vi "Test Phase Retrieval.vi"() -> ()   [LabVIEW 2018]
uses:
  File IO/Image/Tiff/Tiff reader.lvlib
panel:
  out "Function name":string
  out "Python file":path
  out "error out":errorcluster={"status"=FALSE, "code"=0, "source"="XXX"}
  out "Image path":path
  out "Pupil Graph":dbl[][](graph)
  out "Module parent folder":path
  out "Stack sizes":i32[](array[numeric])
  out "Stack Preview":u16[][](graph)
  in  "Slice to preview":i32(slide) scale=0.0..13.0
  # "From python code:"
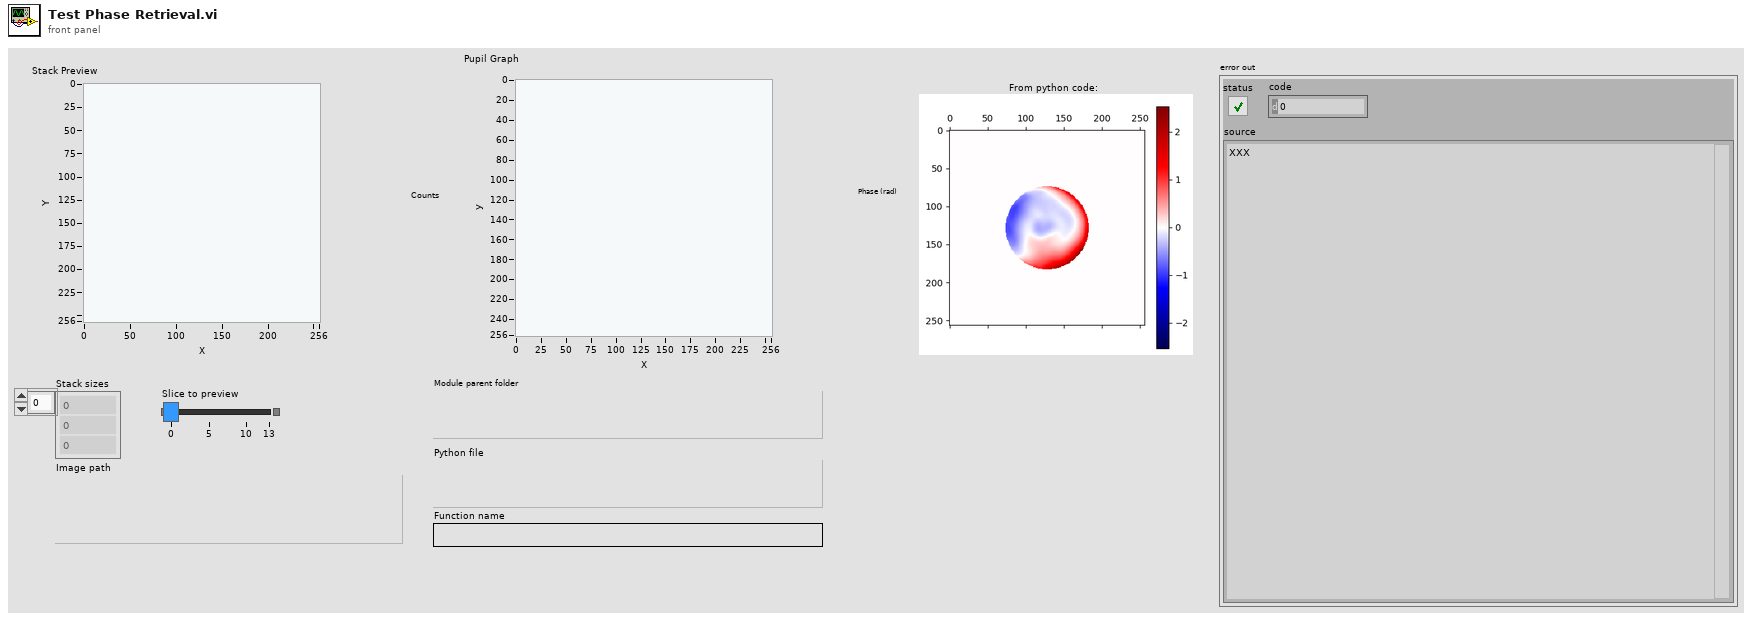
[diagram p1: front panel]
types:
  T1 = enum32{"Gray", "Binary", "Gradient", "Rainbow", "Temperature"}
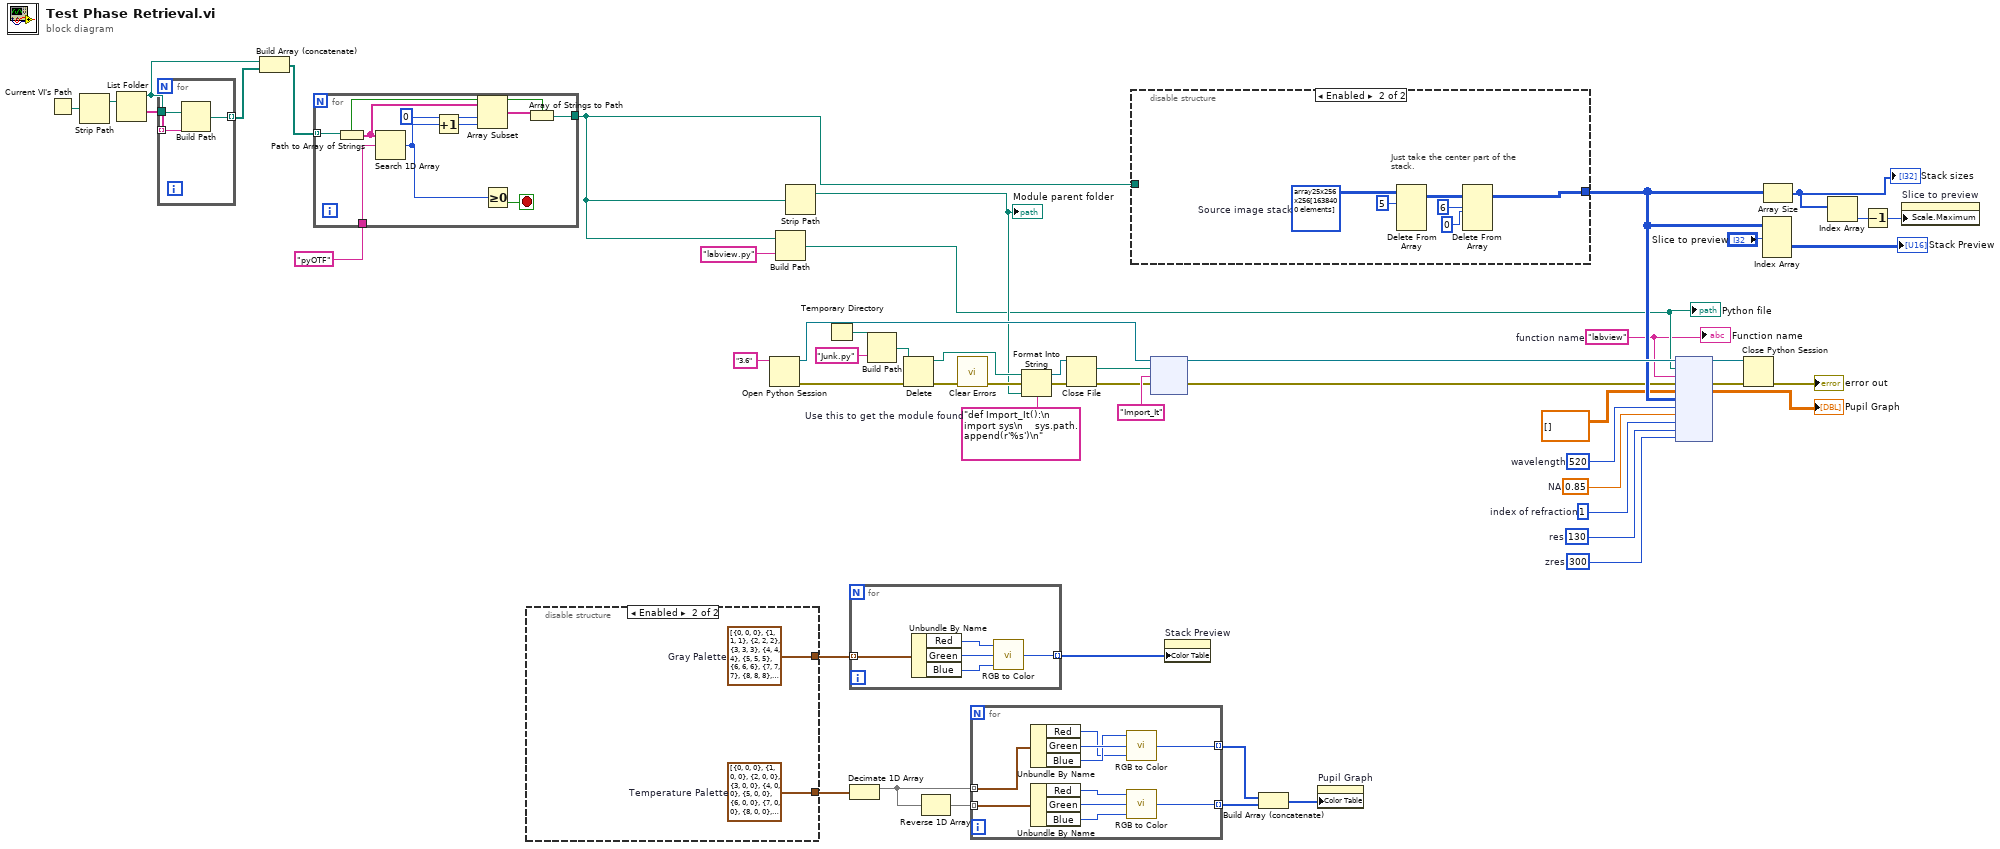
[diagram p0: block diagram]
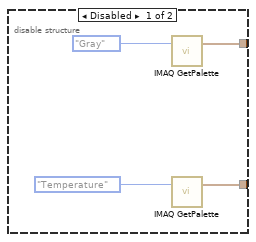
[diagram p2: hidden frame]
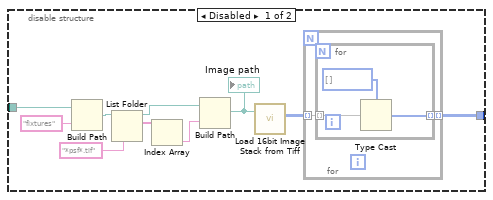
[diagram p3: hidden frame]
diagram:
  w27 = 1  # index of refraction
  w37 = "def Import_It():\n    import sys\n    sys.path.append(r'%s')\n"  # Use this to get the module found
  w26 = 300  # zres
  w25 = 130  # res
  w38 = 0.85  # NA
  w39 = 520  # wavelength
  w2 = "labview"  # function name
  n1 = Current VI's Path() -> (path=w11:path)
  n2 = Strip Path(path=w11) -> (stripped path=w10:path)  [unwired: 1 out]
  n3 = List Folder(path=w10) -> (path out=w7:path, folder names=w9:string[])  [unwired: 3 in, 2 out]
  n4 = for {
    tunnel: w9 -> [w55] mode=indexing
    tunnel: w7 -> [w54]
    tunnel: [w53] -> w8 mode=indexing
    n5 = Build Path(base path=w54, name or relative path=w55) -> (appended path=w53:path)
  }
  n6 = Build Array (concatenate)(w7, w8) -> (w6:path[])
  n7 = for {
    tunnel: w6 -> [w65] mode=indexing
    tunnel: "pyOTF" ("name or relative path") -> [w64]
    tunnel: [w57] -> w4
    stop <- w63 stop-if-true
    n8 = Path to Array of Strings(0:w65) -> (1:w58:bool, 2:w62:string[])
    n9 = Search 1D Array(1D array=w62, element=w64) -> (index of element=w61:i32)  [unwired: 1 in]
    n10 = Increment(x=w61) -> (x+1=w56:i32)
    n11 = Array Subset(array=w62, index=0, length=w56) -> (w59:string[])
    n12 = Greater Or Equal To 0?(x=w61) -> (x >= 0?=w63:bool)
    n13 = Array of Strings to Path(0:w59, 1:w58) -> (2:w57:path)
  }
  n14 = disable-structure shown="Enabled" {
    disable-tunnel: [w68 w71] -> w52
    disable-tunnel: [w66 w70] -> w19
    frame Disabled {
      n15 = call "IMAQ GetPalette"("Palette Number (gray)"=T1."Gray") -> ("Color Palette"=w66:cluster{"Red":u8, "Green":u8, "Blue":u8}[])  [unwired: 4 in, 1 out]
      n16 = call "IMAQ GetPalette"("Palette Number (gray)"=T1."Temperature" ("Palette E")) -> ("Color Palette"=w68:cluster{"Red":u8, "Green":u8, "Blue":u8}[])  [unwired: 4 in, 1 out]
    }
    frame Enabled {
      w70 = cluster{"Red":u8, "Green":u8, "Blue":u8}[] [{"Red"=0, "Green"=0, "Blue"=0}, {"Red"=1, "Green"=1, "Blue"=1}, {"Red"=2, "Green"=2, "Blue"=2}, {"Red"=3, "Green"=3, "Blue"=3}, {"Red"=4, "Green"=4, "Blue"=4}, {"Red"=5, "Green"=5, "Blue"=5}, {"Red"=6, "Green"=6, "Blue"=6}, {"Red"=7, "Green"=7, "Blue"=7}, {"Red"=8, "Green"=8, "Blue"=8}, {"Red"=9, "Green"=9, "Blue"=9}, {"Red"=10, "Green"=10, "Blue"=10}, {"Red"=11, "Green"=11, "Blue"=11}, {"Red"=12, "Green"=12, "Blue"=12}, {"Red"=13, "Green"=13, "Blue"=13}, {"Red"=14, "Green"=14, "Blue"=14}, {"Red"=15, "Green"=15, "Blue"=15}, {"Red"=16, "Green"=16, "Blue"=16}, {"Red"=17, "Green"=17, "Blue"=17}, {"Red"=18, "Green"=18, "Blue"=18}, {"Red"=19, "Green"=19, "Blue"=19}, {"Red"=20, "Green"=20, "Blue"=20}, {"Red"=21, "Green"=21, "Blue"=21}, {"Red"=22, "Green"=22, "Blue"=22}, {"Red"=23, "Green"=23, "Blue"=23}, {"Red"=24, "Green"=24, "Blue"=24}, {"Red"=25, "Green"=25, "Blue"=25}, {"Red"=26, "Green"=26, "Blue"=26}, {"Red"=27, "Green"=27, "Blue"=27}, {"Red"=28, "Green"=28, "Blue"=28}, {"Red"=29, "Green"=29, "Blue"=29}, {"Red"=30, "Green"=30, "Blue"=30}, {"Red"=31, "Green"=31, "Blue"=31}, {"Red"=32, "Green"=32, "Blue"=32}, {"Red"=33, "Green"=33, "Blue"=33}, {"Red"=34, "Green"=34, "Blue"=34}, {"Red"=35, "Green"=35, "Blue"=35}, {"Red"=36, "Green"=36, "Blue"=36}, {"Red"=37, "Green"=37, "Blue"=37}, {"Red"=38, "Green"=38, "Blue"=38}, {"Red"=39, "Green"=39, "Blue"=39}, {"Red"=40, "Green"=40, "Blue"=40}, {"Red"=41, "Green"=41, "Blue"=41}, {"Red"=42, "Green"=42, "Blue"=42}, {"Red"=43, "Green"=43, "Blue"=43}, {"Red"=44, "Green"=44, "Blue"=44}, {"Red"=45, "Green"=45, "Blue"=45}, {"Red"=46, "Green"=46, "Blue"=46}, {"Red"=47, "Green"=47, "Blue"=47}, {"Red"=48, "Green"=48, "Blue"=48}, {"Red"=49, "Green"=49, "Blue"=49}, {"Red"=50, "Green"=50, "Blue"=50}, {"Red"=51, "Green"=51, "Blue"=51}, {"Red"=52, "Green"=52, "Blue"=52}, {"Red"=53, "Green"=53, "Blue"=53}, {"Red"=54, "Green"=54, "Blue"=54}, {"Red"=55, "Green"=55, "Blue"=55}, {"Red"=56, "Green"=56, "Blue"=56}, {"Red"=57, "Green"=57, "Blue"=57}, {"Red"=58, "Green"=58, "Blue"=58}, {"Red"=59, "Green"=59, "Blue"=59}, {"Red"=60, "Green"=60, "Blue"=60}, {"Red"=61, "Green"=61, "Blue"=61}, {"Red"=62, "Green"=62, "Blue"=62}, {"Red"=63, "Green"=63, "Blue"=63}, {"Red"=64, "Green"=64, "Blue"=64}, {"Red"=65, "Green"=65, "Blue"=65}, {"Red"=66, "Green"=66, "Blue"=66}, {"Red"=67, "Green"=67, "Blue"=67}, {"Red"=68, "Green"=68, "Blue"=68}, {"Red"=69, "Green"=69, "Blue"=69}, {"Red"=70, "Green"=70, "Blue"=70}, {"Red"=71, "Green"=71, "Blue"=71}, {"Red"=72, "Green"=72, "Blue"=72}, {"Red"=73, "Green"=73, "Blue"=73}, {"Red"=74, "Green"=74, "Blue"=74}, {"Red"=75, "Green"=75, "Blue"=75}, {"Red"=76, "Green"=76, "Blue"=76}, {"Red"=77, "Green"=77, "Blue"=77}, {"Red"=78, "Green"=78, "Blue"=78}, {"Red"=79, "Green"=79, "Blue"=79}, {"Red"=80, "Green"=80, "Blue"=80}, {"Red"=81, "Green"=81, "Blue"=81}, {"Red"=82, "Green"=82, "Blue"=82}, {"Red"=83, "Green"=83, "Blue"=83}, {"Red"=84, "Green"=84, "Blue"=84}, {"Red"=85, "Green"=85, "Blue"=85}, {"Red"=86, "Green"=86, "Blue"=86}, {"Red"=87, "Green"=87, "Blue"=87}, {"Red"=88, "Green"=88, "Blue"=88}, {"Red"=89, "Green"=89, "Blue"=89}, {"Red"=90, "Green"=90, "Blue"=90}, {"Red"=91, "Green"=91, "Blue"=91}, {"Red"=92, "Green"=92, "Blue"=92}, {"Red"=93, "Green"=93, "Blue"=93}, {"Red"=94, "Green"=94, "Blue"=94}, {"Red"=95, "Green"=95, "Blue"=95}, {"Red"=96, "Green"=96, "Blue"=96}, {"Red"=97, "Green"=97, "Blue"=97}, {"Red"=98, "Green"=98, "Blue"=98}, {"Red"=99, "Green"=99, "Blue"=99}, {"Red"=100, "Green"=100, "Blue"=100}, {"Red"=101, "Green"=101, "Blue"=101}, {"Red"=102, "Green"=102, "Blue"=102}, {"Red"=103, "Green"=103, "Blue"=103}, {"Red"=104, "Green"=104, "Blue"=104}, {"Red"=105, "Green"=105, "Blue"=105}, {"Red"=106, "Green"=106, "Blue"=106}, {"Red"=107, "Green"=107, "Blue"=107}, {"Red"=108, "Green"=108, "Blue"=108}, {"Red"=109, "Green"=109, "Blue"=109}, {"Red"=110, "Green"=110, "Blue"=110}, {"Red"=111, "Green"=111, "Blue"=111}, {"Red"=112, "Green"=112, "Blue"=112}, {"Red"=113, "Green"=113, "Blue"=113}, {"Red"=114, "Green"=114, "Blue"=114}, {"Red"=115, "Green"=115, "Blue"=115}, {"Red"=116, "Green"=116, "Blue"=116}, {"Red"=117, "Green"=117, "Blue"=117}, {"Red"=118, "Green"=118, "Blue"=118}, {"Red"=119, "Green"=119, "Blue"=119}, {"Red"=120, "Green"=120, "Blue"=120}, {"Red"=121, "Green"=121, "Blue"=121}, {"Red"=122, "Green"=122, "Blue"=122}, {"Red"=123, "Green"=123, "Blue"=123}, {"Red"=124, "Green"=124, "Blue"=124}, {"Red"=125, "Green"=125, "Blue"=125}, {"Red"=126, "Green"=126, "Blue"=126}, {"Red"=127, "Green"=127, "Blue"=127}, {"Red"=128, "Green"=128, "Blue"=128}, {"Red"=129, "Green"=129, "Blue"=129}, {"Red"=130, "Green"=130, "Blue"=130}, {"Red"=131, "Green"=131, "Blue"=131}, {"Red"=132, "Green"=132, "Blue"=132}, {"Red"=133, "Green"=133, "Blue"=133}, {"Red"=134, "Green"=134, "Blue"=134}, {"Red"=135, "Green"=135, "Blue"=135}, {"Red"=136, "Green"=136, "Blue"=136}, {"Red"=137, "Green"=137, "Blue"=137}, {"Red"=138, "Green"=138, "Blue"=138}, {"Red"=139, "Green"=139, "Blue"=139}, {"Red"=140, "Green"=140, "Blue"=140}, {"Red"=141, "Green"=141, "Blue"=141}, {"Red"=142, "Green"=142, "Blue"=142}, {"Red"=143, "Green"=143, "Blue"=143}, {"Red"=144, "Green"=144, "Blue"=144}, {"Red"=145, "Green"=145, "Blue"=145}, {"Red"=146, "Green"=146, "Blue"=146}, {"Red"=147, "Green"=147, "Blue"=147}, {"Red"=148, "Green"=148, "Blue"=148}, {"Red"=149, "Green"=149, "Blue"=149}, {"Red"=150, "Green"=150, "Blue"=150}, {"Red"=151, "Green"=151, "Blue"=151}, {"Red"=152, "Green"=152, "Blue"=152}, {"Red"=153, "Green"=153, "Blue"=153}, {"Red"=154, "Green"=154, "Blue"=154}, {"Red"=155, "Green"=155, "Blue"=155}, {"Red"=156, "Green"=156, "Blue"=156}, {"Red"=157, "Green"=157, "Blue"=157}, {"Red"=158, "Green"=158, "Blue"=158}, {"Red"=159, "Green"=159, "Blue"=159}, {"Red"=160, "Green"=160, "Blue"=160}, {"Red"=161, "Green"=161, "Blue"=161}, {"Red"=162, "Green"=162, "Blue"=162}, {"Red"=163, "Green"=163, "Blue"=163}, {"Red"=164, "Green"=164, "Blue"=164}, {"Red"=165, "Green"=165, "Blue"=165}, {"Red"=166, "Green"=166, "Blue"=166}, {"Red"=167, "Green"=167, "Blue"=167}, {"Red"=168, "Green"=168, "Blue"=168}, {"Red"=169, "Green"=169, "Blue"=169}, {"Red"=170, "Green"=170, "Blue"=170}, {"Red"=171, "Green"=171, "Blue"=171}, {"Red"=172, "Green"=172, "Blue"=172}, {"Red"=173, "Green"=173, "Blue"=173}, {"Red"=174, "Green"=174, "Blue"=174}, {"Red"=175, "Green"=175, "Blue"=175}, {"Red"=176, "Green"=176, "Blue"=176}, {"Red"=177, "Green"=177, "Blue"=177}, {"Red"=178, "Green"=178, "Blue"=178}, {"Red"=179, "Green"=179, "Blue"=179}, {"Red"=180, "Green"=180, "Blue"=180}, {"Red"=181, "Green"=181, "Blue"=181}, {"Red"=182, "Green"=182, "Blue"=182}, {"Red"=183, "Green"=183, "Blue"=183}, {"Red"=184, "Green"=184, "Blue"=184}, {"Red"=185, "Green"=185, "Blue"=185}, {"Red"=186, "Green"=186, "Blue"=186}, {"Red"=187, "Green"=187, "Blue"=187}, {"Red"=188, "Green"=188, "Blue"=188}, {"Red"=189, "Green"=189, "Blue"=189}, {"Red"=190, "Green"=190, "Blue"=190}, {"Red"=191, "Green"=191, "Blue"=191}, {"Red"=192, "Green"=192, "Blue"=192}, {"Red"=193, "Green"=193, "Blue"=193}, {"Red"=194, "Green"=194, "Blue"=194}, {"Red"=195, "Green"=195, "Blue"=195}, {"Red"=196, "Green"=196, "Blue"=196}, {"Red"=197, "Green"=197, "Blue"=197}, {"Red"=198, "Green"=198, "Blue"=198}, {"Red"=199, "Green"=199, "Blue"=199}, {"Red"=200, "Green"=200, "Blue"=200}, {"Red"=201, "Green"=201, "Blue"=201}, {"Red"=202, "Green"=202, "Blue"=202}, {"Red"=203, "Green"=203, "Blue"=203}, {"Red"=204, "Green"=204, "Blue"=204}, {"Red"=205, "Green"=205, "Blue"=205}, {"Red"=206, "Green"=206, "Blue"=206}, {"Red"=207, "Green"=207, "Blue"=207}, {"Red"=208, "Green"=208, "Blue"=208}, {"Red"=209, "Green"=209, "Blue"=209}, {"Red"=210, "Green"=210, "Blue"=210}, {"Red"=211, "Green"=211, "Blue"=211}, {"Red"=212, "Green"=212, "Blue"=212}, {"Red"=213, "Green"=213, "Blue"=213}, {"Red"=214, "Green"=214, "Blue"=214}, {"Red"=215, "Green"=215, "Blue"=215}, {"Red"=216, "Green"=216, "Blue"=216}, {"Red"=217, "Green"=217, "Blue"=217}, {"Red"=218, "Green"=218, "Blue"=218}, {"Red"=219, "Green"=219, "Blue"=219}, {"Red"=220, "Green"=220, "Blue"=220}, {"Red"=221, "Green"=221, "Blue"=221}, {"Red"=222, "Green"=222, "Blue"=222}, {"Red"=223, "Green"=223, "Blue"=223}, {"Red"=224, "Green"=224, "Blue"=224}, {"Red"=225, "Green"=225, "Blue"=225}, {"Red"=226, "Green"=226, "Blue"=226}, {"Red"=227, "Green"=227, "Blue"=227}, {"Red"=228, "Green"=228, "Blue"=228}, {"Red"=229, "Green"=229, "Blue"=229}, {"Red"=230, "Green"=230, "Blue"=230}, {"Red"=231, "Green"=231, "Blue"=231}, {"Red"=232, "Green"=232, "Blue"=232}, {"Red"=233, "Green"=233, "Blue"=233}, {"Red"=234, "Green"=234, "Blue"=234}, {"Red"=235, "Green"=235, "Blue"=235}, {"Red"=236, "Green"=236, "Blue"=236}, {"Red"=237, "Green"=237, "Blue"=237}, {"Red"=238, "Green"=238, "Blue"=238}, {"Red"=239, "Green"=239, "Blue"=239}, {"Red"=240, "Green"=240, "Blue"=240}, {"Red"=241, "Green"=241, "Blue"=241}, {"Red"=242, "Green"=242, "Blue"=242}, {"Red"=243, "Green"=243, "Blue"=243}, {"Red"=244, "Green"=244, "Blue"=244}, {"Red"=245, "Green"=245, "Blue"=245}, {"Red"=246, "Green"=246, "Blue"=246}, {"Red"=247, "Green"=247, "Blue"=247}, {"Red"=248, "Green"=248, "Blue"=248}, {"Red"=249, "Green"=249, "Blue"=249}, {"Red"=250, "Green"=250, "Blue"=250}, {"Red"=251, "Green"=251, "Blue"=251}, {"Red"=252, "Green"=252, "Blue"=252}, {"Red"=253, "Green"=253, "Blue"=253}, {"Red"=254, "Green"=254, "Blue"=254}, {"Red"=255, "Green"=255, "Blue"=255}]  # Gray Palette
      w71 = cluster{"Red":u8, "Green":u8, "Blue":u8}[] [{"Red"=0, "Green"=0, "Blue"=0}, {"Red"=1, "Green"=0, "Blue"=0}, {"Red"=2, "Green"=0, "Blue"=0}, {"Red"=3, "Green"=0, "Blue"=0}, {"Red"=4, "Green"=0, "Blue"=0}, {"Red"=5, "Green"=0, "Blue"=0}, {"Red"=6, "Green"=0, "Blue"=0}, {"Red"=7, "Green"=0, "Blue"=0}, {"Red"=8, "Green"=0, "Blue"=0}, {"Red"=9, "Green"=0, "Blue"=0}, {"Red"=10, "Green"=0, "Blue"=0}, {"Red"=11, "Green"=0, "Blue"=0}, {"Red"=12, "Green"=0, "Blue"=0}, {"Red"=13, "Green"=0, "Blue"=0}, {"Red"=14, "Green"=0, "Blue"=0}, {"Red"=15, "Green"=0, "Blue"=0}, {"Red"=16, "Green"=0, "Blue"=0}, {"Red"=17, "Green"=0, "Blue"=0}, {"Red"=18, "Green"=0, "Blue"=0}, {"Red"=19, "Green"=0, "Blue"=0}, {"Red"=20, "Green"=0, "Blue"=0}, {"Red"=21, "Green"=0, "Blue"=0}, {"Red"=22, "Green"=0, "Blue"=0}, {"Red"=23, "Green"=0, "Blue"=0}, {"Red"=24, "Green"=0, "Blue"=0}, {"Red"=25, "Green"=0, "Blue"=0}, {"Red"=26, "Green"=0, "Blue"=0}, {"Red"=27, "Green"=0, "Blue"=0}, {"Red"=28, "Green"=0, "Blue"=0}, {"Red"=29, "Green"=0, "Blue"=0}, {"Red"=30, "Green"=0, "Blue"=0}, {"Red"=31, "Green"=0, "Blue"=0}, {"Red"=32, "Green"=0, "Blue"=0}, {"Red"=33, "Green"=0, "Blue"=0}, {"Red"=34, "Green"=0, "Blue"=0}, {"Red"=35, "Green"=0, "Blue"=0}, {"Red"=36, "Green"=0, "Blue"=0}, {"Red"=37, "Green"=0, "Blue"=0}, {"Red"=38, "Green"=0, "Blue"=0}, {"Red"=39, "Green"=0, "Blue"=0}, {"Red"=40, "Green"=0, "Blue"=0}, {"Red"=41, "Green"=0, "Blue"=0}, {"Red"=42, "Green"=0, "Blue"=0}, {"Red"=43, "Green"=0, "Blue"=0}, {"Red"=44, "Green"=0, "Blue"=0}, {"Red"=45, "Green"=0, "Blue"=0}, {"Red"=46, "Green"=0, "Blue"=0}, {"Red"=47, "Green"=0, "Blue"=0}, {"Red"=48, "Green"=0, "Blue"=0}, {"Red"=49, "Green"=0, "Blue"=0}, {"Red"=50, "Green"=0, "Blue"=0}, {"Red"=51, "Green"=0, "Blue"=0}, {"Red"=52, "Green"=0, "Blue"=0}, {"Red"=53, "Green"=0, "Blue"=0}, {"Red"=54, "Green"=0, "Blue"=0}, {"Red"=55, "Green"=0, "Blue"=0}, {"Red"=56, "Green"=0, "Blue"=0}, {"Red"=57, "Green"=0, "Blue"=0}, {"Red"=58, "Green"=0, "Blue"=0}, {"Red"=59, "Green"=0, "Blue"=0}, {"Red"=60, "Green"=0, "Blue"=0}, {"Red"=61, "Green"=0, "Blue"=0}, {"Red"=62, "Green"=0, "Blue"=0}, {"Red"=63, "Green"=0, "Blue"=0}, {"Red"=64, "Green"=0, "Blue"=0}, {"Red"=65, "Green"=0, "Blue"=0}, {"Red"=66, "Green"=0, "Blue"=0}, {"Red"=67, "Green"=0, "Blue"=0}, {"Red"=68, "Green"=0, "Blue"=0}, {"Red"=69, "Green"=0, "Blue"=0}, {"Red"=70, "Green"=0, "Blue"=0}, {"Red"=71, "Green"=0, "Blue"=0}, {"Red"=72, "Green"=0, "Blue"=0}, {"Red"=73, "Green"=0, "Blue"=0}, {"Red"=74, "Green"=0, "Blue"=0}, {"Red"=75, "Green"=0, "Blue"=0}, {"Red"=76, "Green"=0, "Blue"=0}, {"Red"=77, "Green"=0, "Blue"=0}, {"Red"=78, "Green"=0, "Blue"=0}, {"Red"=79, "Green"=0, "Blue"=0}, {"Red"=80, "Green"=0, "Blue"=0}, {"Red"=81, "Green"=0, "Blue"=0}, {"Red"=82, "Green"=0, "Blue"=0}, {"Red"=83, "Green"=0, "Blue"=0}, {"Red"=84, "Green"=0, "Blue"=0}, {"Red"=85, "Green"=0, "Blue"=0}, {"Red"=86, "Green"=0, "Blue"=0}, {"Red"=87, "Green"=0, "Blue"=0}, {"Red"=88, "Green"=0, "Blue"=0}, {"Red"=89, "Green"=0, "Blue"=0}, {"Red"=90, "Green"=0, "Blue"=0}, {"Red"=91, "Green"=0, "Blue"=0}, {"Red"=92, "Green"=0, "Blue"=0}, {"Red"=93, "Green"=0, "Blue"=0}, {"Red"=94, "Green"=0, "Blue"=0}, {"Red"=95, "Green"=0, "Blue"=0}, {"Red"=96, "Green"=0, "Blue"=0}, {"Red"=97, "Green"=0, "Blue"=0}, {"Red"=98, "Green"=0, "Blue"=0}, {"Red"=99, "Green"=0, "Blue"=0}, {"Red"=100, "Green"=0, "Blue"=0}, {"Red"=101, "Green"=0, "Blue"=0}, {"Red"=102, "Green"=0, "Blue"=0}, {"Red"=103, "Green"=0, "Blue"=0}, {"Red"=104, "Green"=0, "Blue"=0}, {"Red"=105, "Green"=1, "Blue"=0}, {"Red"=106, "Green"=3, "Blue"=0}, {"Red"=107, "Green"=5, "Blue"=0}, {"Red"=108, "Green"=6, "Blue"=0}, {"Red"=109, "Green"=8, "Blue"=0}, {"Red"=110, "Green"=10, "Blue"=0}, {"Red"=111, "Green"=11, "Blue"=0}, {"Red"=112, "Green"=13, "Blue"=0}, {"Red"=113, "Green"=15, "Blue"=0}, {"Red"=114, "Green"=16, "Blue"=0}, {"Red"=115, "Green"=18, "Blue"=0}, {"Red"=116, "Green"=20, "Blue"=0}, {"Red"=117, "Green"=21, "Blue"=0}, {"Red"=118, "Green"=23, "Blue"=0}, {"Red"=119, "Green"=25, "Blue"=0}, {"Red"=120, "Green"=27, "Blue"=0}, {"Red"=121, "Green"=28, "Blue"=0}, {"Red"=122, "Green"=30, "Blue"=0}, {"Red"=123, "Green"=32, "Blue"=0}, {"Red"=124, "Green"=33, "Blue"=0}, {"Red"=125, "Green"=35, "Blue"=0}, {"Red"=126, "Green"=37, "Blue"=0}, {"Red"=127, "Green"=38, "Blue"=0}, {"Red"=128, "Green"=40, "Blue"=0}, {"Red"=129, "Green"=42, "Blue"=0}, {"Red"=130, "Green"=43, "Blue"=0}, {"Red"=131, "Green"=45, "Blue"=0}, {"Red"=132, "Green"=47, "Blue"=0}, {"Red"=133, "Green"=48, "Blue"=0}, {"Red"=134, "Green"=50, "Blue"=0}, {"Red"=135, "Green"=52, "Blue"=0}, {"Red"=136, "Green"=54, "Blue"=0}, {"Red"=137, "Green"=55, "Blue"=0}, {"Red"=138, "Green"=57, "Blue"=0}, {"Red"=139, "Green"=59, "Blue"=0}, {"Red"=140, "Green"=60, "Blue"=0}, {"Red"=141, "Green"=62, "Blue"=0}, {"Red"=142, "Green"=64, "Blue"=0}, {"Red"=143, "Green"=65, "Blue"=2}, {"Red"=144, "Green"=67, "Blue"=4}, {"Red"=145, "Green"=69, "Blue"=6}, {"Red"=146, "Green"=70, "Blue"=9}, {"Red"=147, "Green"=72, "Blue"=11}, {"Red"=148, "Green"=74, "Blue"=13}, {"Red"=149, "Green"=75, "Blue"=15}, {"Red"=150, "Green"=77, "Blue"=18}, {"Red"=151, "Green"=79, "Blue"=20}, {"Red"=152, "Green"=81, "Blue"=22}, {"Red"=153, "Green"=82, "Blue"=24}, {"Red"=154, "Green"=84, "Blue"=27}, {"Red"=155, "Green"=86, "Blue"=29}, {"Red"=156, "Green"=87, "Blue"=31}, {"Red"=157, "Green"=89, "Blue"=33}, {"Red"=158, "Green"=91, "Blue"=36}, {"Red"=159, "Green"=92, "Blue"=38}, {"Red"=160, "Green"=94, "Blue"=40}, {"Red"=161, "Green"=96, "Blue"=42}, {"Red"=162, "Green"=97, "Blue"=45}, {"Red"=163, "Green"=99, "Blue"=47}, {"Red"=164, "Green"=101, "Blue"=49}, {"Red"=165, "Green"=103, "Blue"=51}, {"Red"=166, "Green"=104, "Blue"=54}, {"Red"=167, "Green"=106, "Blue"=56}, {"Red"=168, "Green"=108, "Blue"=58}, {"Red"=169, "Green"=109, "Blue"=60}, {"Red"=170, "Green"=111, "Blue"=63}, {"Red"=171, "Green"=113, "Blue"=65}, {"Red"=172, "Green"=114, "Blue"=67}, {"Red"=173, "Green"=116, "Blue"=69}, {"Red"=174, "Green"=118, "Blue"=72}, {"Red"=175, "Green"=119, "Blue"=74}, {"Red"=176, "Green"=121, "Blue"=76}, {"Red"=177, "Green"=123, "Blue"=78}, {"Red"=178, "Green"=124, "Blue"=81}, {"Red"=179, "Green"=126, "Blue"=83}, {"Red"=180, "Green"=128, "Blue"=85}, {"Red"=181, "Green"=130, "Blue"=88}, {"Red"=182, "Green"=131, "Blue"=90}, {"Red"=183, "Green"=133, "Blue"=92}, {"Red"=184, "Green"=135, "Blue"=94}, {"Red"=185, "Green"=136, "Blue"=97}, {"Red"=186, "Green"=138, "Blue"=99}, {"Red"=187, "Green"=140, "Blue"=101}, {"Red"=188, "Green"=141, "Blue"=103}, {"Red"=189, "Green"=143, "Blue"=106}, {"Red"=190, "Green"=145, "Blue"=108}, {"Red"=191, "Green"=146, "Blue"=110}, {"Red"=192, "Green"=148, "Blue"=112}, {"Red"=193, "Green"=150, "Blue"=115}, {"Red"=194, "Green"=151, "Blue"=117}, {"Red"=195, "Green"=153, "Blue"=119}, {"Red"=196, "Green"=155, "Blue"=121}, {"Red"=197, "Green"=157, "Blue"=124}, {"Red"=198, "Green"=158, "Blue"=126}, {"Red"=199, "Green"=160, "Blue"=128}, {"Red"=200, "Green"=162, "Blue"=130}, {"Red"=201, "Green"=163, "Blue"=133}, {"Red"=202, "Green"=165, "Blue"=135}, {"Red"=203, "Green"=167, "Blue"=137}, {"Red"=204, "Green"=168, "Blue"=139}, {"Red"=205, "Green"=170, "Blue"=142}, {"Red"=206, "Green"=172, "Blue"=144}, {"Red"=207, "Green"=173, "Blue"=146}, {"Red"=208, "Green"=175, "Blue"=148}, {"Red"=209, "Green"=177, "Blue"=151}, {"Red"=210, "Green"=179, "Blue"=153}, {"Red"=211, "Green"=180, "Blue"=155}, {"Red"=212, "Green"=182, "Blue"=157}, {"Red"=213, "Green"=184, "Blue"=160}, {"Red"=214, "Green"=185, "Blue"=162}, {"Red"=215, "Green"=187, "Blue"=164}, {"Red"=216, "Green"=189, "Blue"=166}, {"Red"=217, "Green"=190, "Blue"=169}, {"Red"=218, "Green"=192, "Blue"=171}, {"Red"=219, "Green"=194, "Blue"=173}, {"Red"=220, "Green"=195, "Blue"=176}, {"Red"=221, "Green"=197, "Blue"=178}, {"Red"=222, "Green"=199, "Blue"=180}, {"Red"=223, "Green"=200, "Blue"=182}, {"Red"=224, "Green"=202, "Blue"=185}, {"Red"=225, "Green"=204, "Blue"=187}, {"Red"=226, "Green"=206, "Blue"=189}, {"Red"=227, "Green"=207, "Blue"=191}, {"Red"=228, "Green"=209, "Blue"=194}, {"Red"=229, "Green"=211, "Blue"=196}, {"Red"=230, "Green"=212, "Blue"=198}, {"Red"=231, "Green"=214, "Blue"=200}, {"Red"=232, "Green"=216, "Blue"=203}, {"Red"=233, "Green"=217, "Blue"=205}, {"Red"=234, "Green"=219, "Blue"=207}, {"Red"=235, "Green"=221, "Blue"=209}, {"Red"=236, "Green"=222, "Blue"=212}, {"Red"=237, "Green"=224, "Blue"=214}, {"Red"=238, "Green"=226, "Blue"=216}, {"Red"=239, "Green"=227, "Blue"=218}, {"Red"=240, "Green"=229, "Blue"=221}, {"Red"=241, "Green"=231, "Blue"=223}, {"Red"=242, "Green"=233, "Blue"=225}, {"Red"=243, "Green"=234, "Blue"=227}, {"Red"=244, "Green"=236, "Blue"=230}, {"Red"=245, "Green"=238, "Blue"=232}, {"Red"=246, "Green"=239, "Blue"=234}, {"Red"=247, "Green"=241, "Blue"=236}, {"Red"=248, "Green"=243, "Blue"=239}, {"Red"=249, "Green"=244, "Blue"=241}, {"Red"=250, "Green"=246, "Blue"=243}, {"Red"=251, "Green"=248, "Blue"=245}, {"Red"=252, "Green"=249, "Blue"=248}, {"Red"=253, "Green"=251, "Blue"=250}, {"Red"=254, "Green"=253, "Blue"=252}, {"Red"=255, "Green"=255, "Blue"=255}]  # Temperature Palette
    }
  }
  n17 = Open Python Session(python version="3.6" ("Python version")) -> (session out=w36:refnum<k35>, error out=w20:errorcluster)  [unwired: 2 in]
  n18 = Build Path(base path=w4, name or relative path="labview.py") -> (appended path=w3:path)
  "Python file" <- w3
  n19 = Strip Path(path=w4) -> (stripped path=w12:path)  [unwired: 1 out]
  "Module parent folder" <- w12
  n20 = Temporary Directory() -> (w15:path)
  n21 = for {
    tunnel: w19 -> [w73] mode=indexing
    tunnel: [w72] -> w1 mode=indexing
    n22 = Unbundle By Name(w73) -> ("Red"=w74:u8, "Green"=w75:u8, "Blue"=w76:u8)
    n23 = call <vilib>:"RGB to Color.vi"("B"=w76, "G"=w75, "R"=w74) -> ("Color"=w72:u32)
  }
  n24 = Decimate 1D Array(w52) -> (w51:cluster{"Red":u8, "Green":u8, "Blue":u8}[])  [unwired: 1 out]
  n25 = Build Path(base path=w15, name or relative path="Junk.py") -> (appended path=w14:path)
  n26 = Delete(path (use dialog)=w14) -> (deleted path=w30:path, error out=w29:errorcluster)  [unwired: 4 in, 1 out]
  n27 = Reverse 1D Array(array=w51) -> (reversed array=w47:cluster{"Red":u8, "Green":u8, "Blue":u8}[])
  n28 = call <vilib>:"Clear Errors.vi"("error in (no error)"=w29) -> ("error out"=w28:errorcluster)  [unwired: 5 in, 1 out]
  n29 = for {
    tunnel: w47 -> [w83] mode=indexing
    tunnel: [w82] -> w50 mode=indexing
    tunnel: w51 -> [w80] mode=indexing
    tunnel: [w77] -> w49 mode=indexing
    n30 = Unbundle By Name(w80) -> ("Red"=w78:u8, "Green"=w81:u8, "Blue"=w79:u8)
    n31 = Unbundle By Name(w83) -> ("Red"=w86:u8, "Green"=w85:u8, "Blue"=w84:u8)
    n32 = call <vilib>:"RGB to Color.vi"("B"=w78, "G"=w81, "R"=w79) -> ("Color"=w77:u32)
    n33 = call <vilib>:"RGB to Color.vi"("B"=w84, "G"=w85, "R"=w86) -> ("Color"=w82:u32)
  }
  n34 = Format Into String(format string=w37, initial string=w30, error in=w28, w12) -> (resulting string=w34:refnum<file>, error out=w33:errorcluster)
  n35 = Close File(refnum=w34, error in=w33) -> (path=w32:path)  [unwired: 1 out]
  n36 = disable-structure shown="Enabled" {
    disable-tunnel: w4 -> [w90 _]
    disable-tunnel: [w88 w102] -> w24
    frame Disabled {
      n37 = Build Path(base path=w90, name or relative path="fixtures") -> (appended path=w95:path)
      n38 = List Folder(path=w95, pattern="*psf*.tif") -> (path out=w92:path, filenames=w93:string[])  [unwired: 2 in, 2 out]
      n39 = Index Array(array=w93) -> (element=w91:string)  [unwired: 1 in]
      n40 = Build Path(base path=w92, name or relative path=w91) -> (appended path=w89:path)
      "Image path" <- w89
      n41 = call "Load 16bit Image Stack from Tiff.vi"("path to TIFF file"=w89) -> ("I16"=w87:i16[][][])  [unwired: 4 in, 2 out]
      n42 = for {
        tunnel: w87 -> [w98] mode=indexing
        tunnel: [w97] -> w88 mode=indexing
        n43 = for {
          tunnel: w98 -> [w101] mode=indexing
          tunnel: [w99] -> w97 mode=indexing
          n44 = Type Cast(type=u16[] [] ("Gray8"), x=w101) -> (*(type *) &x=w99:u16[])
        }
      }
    }
    frame Enabled {
      w107 = u16[][][] array25x256x256[1638400 elements]  # Source image stack
      # "Just take the center part of the \nstack."
      n45 = Delete From Array(array=w107, length=5) -> (array with subset deleted=w105:u16[][][])  [unwired: 3 in, 1 out]
      n46 = Delete From Array(array=w105, length=6, index (dim 0)=0 ("index (page)")) -> (array with subset deleted=w102:u16[][][])  [unwired: 2 in, 1 out]
    }
  }
  n47 = node(w36, w32, "Import_It" ("function name"), w20) -> (w35:refnum<k35>, w16:errorcluster)  [unwired: 2 in, 2 out]
  n48 = property on="Stack Preview" class="IntGraph (strict)"("Color Table"=w1) -> ()  [unwired: 2 in, 2 out]
  n49 = Build Array (concatenate)(w49, w50) -> (w48:u32[])
  n50 = property on="Pupil Graph" class="IntGraph (strict)"("Color Table"=w48) -> ()  [unwired: 2 in, 2 out]
  n51 = node(w35, w3, w2, w16, dbl[][] [] ("Gray8"), w24, w39, w38, w27, w25, w26) -> (w40:refnum<k35>, w17:errorcluster, →"Pupil Graph":dbl[][])  [unwired: 6 in, 2 out]
  n52 = Close Python Session(session in=w40, error in=w17) -> (11:→"error out":errorcluster)
  n53 = Index Array(array=w24, index (dim 0)="Slice to preview") -> (element=→"Stack Preview":u16[][])  [unwired: 2 in]
  n54 = Array Size(array=w24) -> (size(s)=w44:i32[])
  "Stack sizes" <- w44
  n55 = Index Array(array=w44) -> (element=w43:i32)  [unwired: 1 in]
  n56 = Decrement(x=w43) -> (x-1=w42:i32)
  n57 = property on="Slice to preview" class="Slide (strict)"("Scale.Maximum"=w42) -> ()  [unwired: 2 in, 2 out]
  "Function name" <- w2
